vi "AMI1700eth_close.vi"(8 "error in":errorcluster, 11 "conn_id":refnum<k5>) -> (0 "error out":errorcluster, 3 "conn_id_out":refnum<k5>)   [LabVIEW 2019]
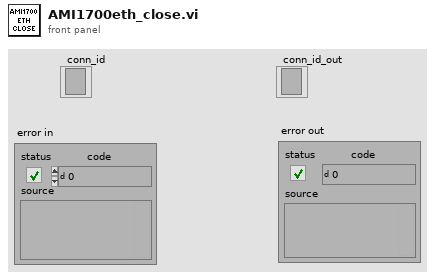
[diagram p1: front panel]
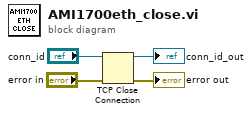
[diagram p0: block diagram]
diagram:
  n1 = TCP Close Connection(connection ID="conn_id", error in (no error)="error in") -> (connection ID out=→"conn_id_out":refnum<k5>, error out=→"error out":errorcluster)  [unwired: 1 in]
